vi "Teleop.vi"(10 "Match Info":T1={"Autonomous Elapsed Seconds"=0.0, "TeleOp Elapsed Seconds"=0.0, "Disabled Elapsed Seconds"=0.0, "Visited Autonomous"=FALSE, "Visited TeleOp"=FALSE, "Visited Disabled"=FALSE, "Autonomous Settings"={"Autonomous Style"=enum."Independent", "VI Refnum"=refnum}}, 11 "Call Context":T2) -> ()   [LabVIEW 2023]
doc: "This VI is called for each enabled TeleOp packet received from the DS. It is typically used to read from joysticks and other inputs and update I/O or setpoints for timed control loops. It should complete and return within 20 milliseconds or risk missing DS packets."
uses:
  <vilib>/Rock Robotics/WPI/DriverStation/WPI_DriverStationDerivedRobotMode.ctl
  <vilib>/Rock Robotics/WPI/DriverStation/WPI_DriverStationMatch Info.ctl
  <vilib>/Rock Robotics/WPI/Joystick/XBox Buttons Indexer.ctl
  <vilib>/Rock Robotics/WPI/ThirdParty/JAS_Junk/TrajLib/Conv_Deg_Radians.vi
  <vilib>/Rock Robotics/WPI/ThirdParty/JAS_Junk/TrajLib/Rotation2d_CreateAngle.vi
  <vilib>/Rock Robotics/WPI/ThirdParty/JAS_Junk/TrajLib/Rotation2d_GetCos.vi
  <vilib>/Rock Robotics/WPI/ThirdParty/JAS_Junk/TrajLib/Rotation2d_GetSin.vi
  <vilib>/Rock Robotics/WPI/ThirdParty/JAS_Junk/TrajLib/ChassisSpeeds_New.vi
  <vilib>/Rock Robotics/WPI/Utilities/WPI_GetSetVariantRefNum.vi
  <vilib>/Rock Robotics/Network Tables/NT Write Numeric Array.vi
  <vilib>/Rock Robotics/Network Tables/NT Write Boolean Array.vi
  <vilib>/Rock Robotics/WPI/ThirdParty/JAS_Junk/TrajLib/TypeDef/CHASSIS_SPEEDS.ctl
  Swerve/Implementation/Swerve Operations.ctl
  <vilib>/Rock Robotics/WPI/ThirdParty/JAS_Junk/TrajLib/Trajectory_Library.lvlib
  Swerve/Implementation/Swerve Setpoints.ctl
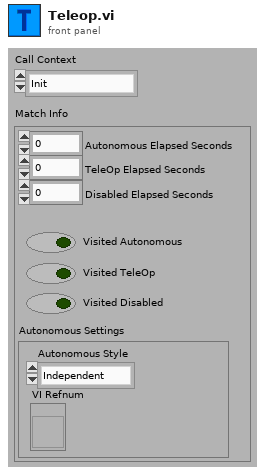
[diagram p1: front panel]
types:
  T1 = typedef "WPI_DriverStationMatch Info.ctl" = cluster{"Autonomous Elapsed Seconds":dbl, "TeleOp Elapsed Seconds":dbl, "Disabled Elapsed Seconds":dbl, "Visited Autonomous":bool, "Visited TeleOp":bool, "Visited Disabled":bool, "Autonomous Settings":cluster{"Autonomous Style":enum16{"Iterative", "Independent"}, "VI Refnum":refnum<vi>}}
  T2 = typedef "WPI_DriverStationDerivedRobotMode.ctl" = enum16{"Init", "Execute", "Stop"}
  T3 = typedef "XBox Buttons Indexer.ctl" = enum16{"A", "B", "X", "Y", "Left Bumper", "Right Bumper", "Back", "Start", "Left Joystick", "Right Joystick"}
  T4 = typedef "Swerve Operations.ctl" = enum16{"Reserve", "Read Current", "Immediate", "Joystick Drive"}
  T5 = typedef "Swerve Setpoints.ctl" = cluster{"Operation":T4, "CHASSIS":T6}
  T6 = typedef "Trajectory_Library.lvlib/CHASSIS_SPEEDS.ctl" = cluster{"vX":dbl, "vY":dbl, "vOmega":dbl}
  T7 = typedef "WPI_JoystickDevRef.ctl" = cluster{"Device":T8}
  T8 = typedef "WPI_JoystickDeviceEnum.ctl" = enum16{"USB 0", "USB 1", "USB 2", "USB 3", "USB 4", "USB 5"}
  T9 = typedef "ADIS16470 Device Reference.ctl" = cluster{"DevStatus":errorcluster, "Hardware Config":T10, "Calibration Complete":refnum<notifier>, "Status Reference":refnum<data-value>, "Data Reference":refnum<data-value>, "Sychronous Process VI":T14, "Cmd FIFO":refnum<k33>, "Source":T15, "Data FIFO":refnum<k33>, "Calibration Time (ms)":u32, "Data Reference":refnum<data-value>}
  T10 = typedef "ADIS16470 Hardware Configuration.ctl" = cluster{"SPI Clock Rate (Hz)":dbl, "IMU SPI Mode (3)":T11, "IMU Reset Pin":T12, "IMU SPI Bus":T13, "IMU Data Ready Pin":T12, "Stall Config":cluster{"Pow2BytesPerRead":u8, "StallTicks":u16, "CsToSclkTicks":u8}}
  T11 = typedef "WPI_SPIMode.ctl" = enum16{"Mode 0 (Clk Idle Low,Sample on Leading)", "Mode 1 (Clk Idle Low,Sample on Trailing)", "Mode 2 (Clk Idle High,Sample on Leading)", "Mode 3 (Clk Idle High,Sample on Trailing)"}
  T12 = typedef "FPGA_DIOChannel.ctl" = enum8{"DIO 0", "DIO 1", "DIO 2", "DIO 3", "DIO 4", "DIO 5", "DIO 6", "DIO 7", "DIO 8", "DIO 9", "DIO MXP 0", "DIO MXP 1", "DIO MXP 2", "DIO MXP 3", "DIO MXP 4", "DIO MXP 5", "DIO MXP 6", "DIO MXP 7", "DIO MXP 8", "DIO MXP 9", "DIO MXP 10", "DIO MXP 11", "DIO MXP 12", "DIO MXP 13", "DIO MXP 14", "DIO MXP 15", "SPI Port CS1", "SPI Port CS2", "SPI Port CS3", "SPI Port MISO", "SPI Port MOSI", "Invalid"}
  T13 = typedef "spi_bus.ctl" = enum16{"SPI On-Board, CS0", "SPI On-Board, CS1", "SPI On-Board, CS2", "SPI On-Board, CS3", "SPI MXP", "Invalid"}
  T14 = typedef "ADIS16470 Process.ctl" = refnum<vi>
  T15 = typedef "FPGA_CounterEncoderSourceConvertionLVSourceType.ctl" = cluster{"DevStatus":errorcluster, "AnalogTriggerMode?":bool, "DigitalMode":cluster{"DIO Channel":T16}, "AnalogTriggerMode":cluster{"AnalogTriggerIndex":T17, "OutputType":T18}}
  T16 = typedef "FPGA_DIODigitalSourceChannel.ctl" = enum8{"DIO 0", "DIO 1", "DIO 2", "DIO 3", "DIO 4", "DIO 5", "DIO 6", "DIO 7", "DIO 8", "DIO 9", "DIO MXP 0", "DIO MXP 1", "DIO MXP 2", "DIO MXP 3", "DIO MXP 4", "DIO MXP 5", "DIO MXP 6", "DIO MXP 7", "DIO MXP 8", "DIO MXP 9", "DIO MXP 10", "DIO MXP 11", "DIO MXP 12", "DIO MXP 13", "DIO MXP 14", "DIO MXP 15", "SPI Port CS1", "SPI Port CS2", "SPI Port CS3", "SPI Port MISO", "SPI Port MOSI", "Disabled"}
  T17 = typedef "FPGA_AnalogTriggerIndex.ctl" = enum8{"Trig 0", "Trig 1", "Trig 2", "Trig 3", "Trig 4", "Trig 5", "Trig 6", "Trig 7", "Invalid"}
  T18 = typedef "FPGA_AnalogTriggerOutType.ctl" = enum16{"InWindow", "TriggerState", "Rising", "Falling"}
  T19 = typedef "ADIS16470 Data.ctl" = cluster{"XAngle":dbl, "YAngle":dbl, "ZAngle":dbl}
  T20 = typedef "Trajectory_Library.lvlib/ROTATION2D.ctl" = cluster{"VALUE":dbl, "COS":dbl, "SIN":dbl}
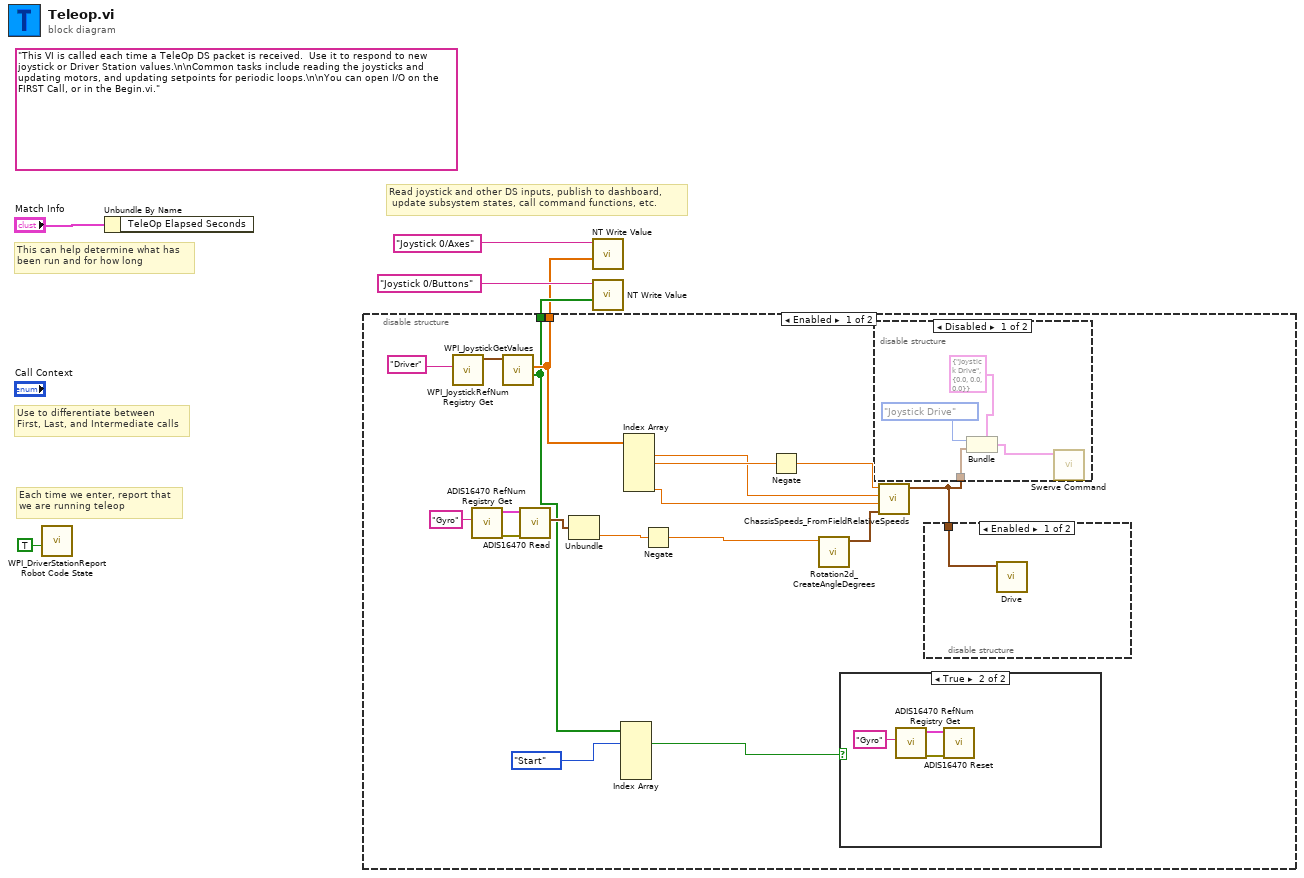
[diagram p0: block diagram]
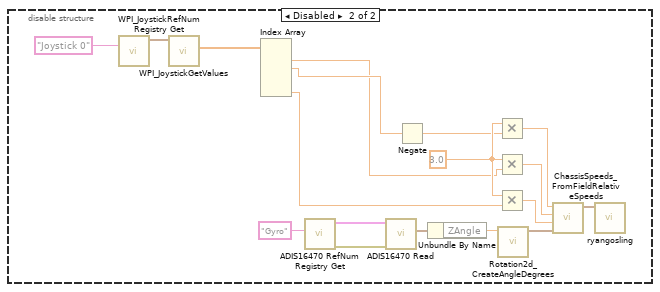
[diagram p5: hidden frame]
diagram:
  (unwired) "This VI is called each time a TeleOp DS packet is received.  Use it to respond to new joystick or Driver Station values.\n\nCommon tasks include reading the joysticks and updating motors, and updating setpoints for periodic loops.\n\nYou can open I/O on the FIRST Call, or in the Begin.vi."
  # "Read joystick and other DS inputs, publish to dashboard,\n update subsystem states, call command functions, etc."
  # "Each time we enter, report that\nwe are running teleop"
  # "Use to differentiate between\nFirst, Last, and Intermediate calls"
  # "This can help determine what has\nbeen run and for how long"
  n1 = call <vilib>:"WPI_DriverStationReport Robot Code State.vi"("TeleOp"=TRUE ("Autonomous")) -> ()  [unwired: 10 in, 1 out]
  n2 = Unbundle By Name("Match Info") -> ()  [unwired: 1 out]
  n3 = disable-structure shown="Enabled" {
    disable-tunnel: [w9 _] -> w3
    disable-tunnel: [w22 _] -> w1
    frame Enabled {
      n4 = call <vilib>:"WPI_JoystickRefNum Registry Get.vi"("refnum name"="Driver") -> ("JoystickDevRef"=w23:T7)  [unwired: 1 in, 9 out]
      n5 = call <vilib>:"ADIS16470 RefNum Registry Get.vi"("refnum name"="Gyro") -> ("error out"=w20:errorcluster, "ADIS16470DevRef out"=w21:T9)  [unwired: 9 in]
      n6 = call <vilib>:"WPI_JoystickGetValues.vi"("JoystickDevRef"=w23) -> ("Buttons"=w9:bool[], "Axes"=w22:dbl[])  [unwired: 6 in, 3 out]
      n7 = call <vilib>:"ADIS16470 Read.vi"("error in (no error)"=w20, "ADIS16470DevRef"=w21) -> ("ADIS16470 Value"=w18:T19)  [unwired: 6 in, 3 out]
      n8 = Unbundle(w18) -> ("ZAngle"=w12:dbl)  [unwired: 2 out]
      n9 = Index Array(array=w9, index #1=XBox_Buttons_Indexer."Start" ("XBox Buttons")) -> (element #1=w7:bool)  [unwired: 4 in, 4 out]
      n10 = Index Array(array=w22) -> (element #1=w15:dbl, element #2=w16:dbl, element #5=w14:dbl)  [unwired: 5 in, 2 out]
      n11 = Negate(x=w12) -> (-x=w11:dbl)
      n12 = Negate(x=w16) -> (-x=w10:dbl)
      n13 = call <vilib>:"Rotation2d_CreateAngleDegrees.vi"("Angle_Degrees"=w11) -> ("ROTATION"=w17:T20)  [unwired: 10 in]
      n14 = case shown="True" w7 {
        frame False {
        }
        frame True {
          n15 = call <vilib>:"ADIS16470 RefNum Registry Get.vi"("refnum name"="Gyro") -> ("error out"=w26:errorcluster, "ADIS16470DevRef out"=w25:T9)  [unwired: 9 in]
          n16 = call <vilib>:"ADIS16470 Reset.vi"("error in (no error)"=w26, "ADIS16470DevRef"=w25) -> ()  [unwired: 8 in, 2 out]
        }
      }
      n17 = call <vilib>:"ChassisSpeeds_FromFieldRelativeSpeeds.vi"("RobotAngle"=w17, "Omega"=w14, "vY"=w15, "vX"=w10) -> ("CHASSIS"=w13:T6)  [unwired: 7 in]
      n18 = disable-structure shown="Disabled" {
        disable-tunnel: w13 -> [w29 _]
        frame Disabled {
          n19 = Bundle(cluster=T5 {"Operation"=enum."Joystick Drive", "CHASSIS"={"vX"=0.0, "vY"=0.0, "vOmega"=0.0}} ("SubSystem Data"), "Operation"=Swerve_Operations."Joystick Drive", "CHASSIS"=w29) -> (w31:T5)
          n20 = call "Swerve Command.vi"("SubSystem Data"=w31) -> ()  [unwired: 10 in, 1 out]
        }
        frame Enabled {
        }
      }
      n21 = disable-structure shown="Enabled" {
        disable-tunnel: w13 -> [w28 _]
        frame Enabled {
          n22 = call "Drive.vi"("CHASSIS"=w28) -> ()  [unwired: 9 in, 2 out]
        }
        frame Disabled {
        }
      }
    }
    frame Disabled {
      w39 = 3.0 ("x")
      n23 = call <vilib>:"WPI_JoystickRefNum Registry Get.vi"("refnum name"="Joystick 0") -> ("JoystickDevRef"=w50:T7)  [unwired: 1 in, 9 out]
      n24 = call <vilib>:"WPI_JoystickGetValues.vi"("JoystickDevRef"=w50) -> ("Axes"=w49:dbl[])  [unwired: 6 in, 4 out]
      n25 = Index Array(array=w49) -> (element #1=w37:dbl, element #2=w38:dbl, element #5=w36:dbl)  [unwired: 5 in, 2 out]
      n26 = call <vilib>:"ADIS16470 RefNum Registry Get.vi"("refnum name"="Gyro") -> ("error out"=w46:errorcluster, "ADIS16470DevRef out"=w43:T9)  [unwired: 9 in]
      n27 = call <vilib>:"ADIS16470 Read.vi"("error in (no error)"=w46, "ADIS16470DevRef"=w43) -> ("ADIS16470 Value"=w47:T19)  [unwired: 6 in, 3 out]
      n28 = Negate(x=w38) -> (-x=w35:dbl)
      n29 = Unbundle By Name(w47) -> ("ZAngle"=w33:dbl)
      n30 = Multiply(x=w39, y=w35) -> (x*y=w40:dbl)
      n31 = Multiply(x=w39, y=w37) -> (x*y=w41:dbl)
      n32 = Multiply(x=w39, y=w36) -> (x*y=w42:dbl)
      n33 = call <vilib>:"Rotation2d_CreateAngleDegrees.vi"("Angle_Degrees"=w33) -> ("ROTATION"=w44:T20)  [unwired: 10 in]
      n34 = call <vilib>:"ChassisSpeeds_FromFieldRelativeSpeeds.vi"("RobotAngle"=w44, "Omega"=w42, "vY"=w41, "vX"=w40) -> ("CHASSIS"=w48:T6)  [unwired: 7 in]
      n35 = call "ryangosling.vi"("CHASSIS"=w48) -> ()  [unwired: 9 in, 2 out]
    }
  }
  n36 = call-poly <vilib>:"NT Write Value.vi"("value"=w1, "name"="Joystick 0/Axes" ("Name")) -> ()  [unwired: 9 in, 1 out]
  n37 = call-poly <vilib>:"NT Write Value.vi"("value"=w3, "name"="Joystick 0/Buttons" ("Name")) -> ()  [unwired: 9 in, 1 out]
